vi "Exchange AI.vi"(8 "error in (no error)":errorcluster, 10 "AIP in":dbl[][](array[numeric]), 11 "AIP DVR":refnum<data-value>) -> (0 "error out":errorcluster, 2 "AIP out":dbl[][](array[numeric]), 3 "AIP DVR out":refnum<data-value>)   [LabVIEW 2019, in "Inputs.lvlib"]
uses:
  Inputs.lvlib
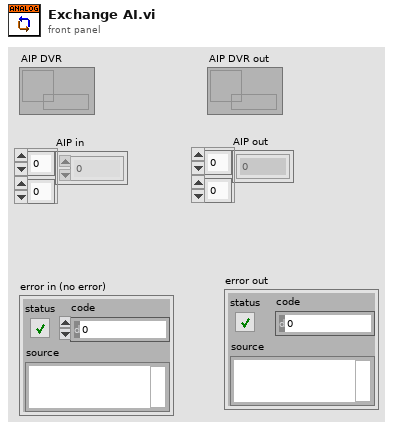
[diagram p1: front panel]
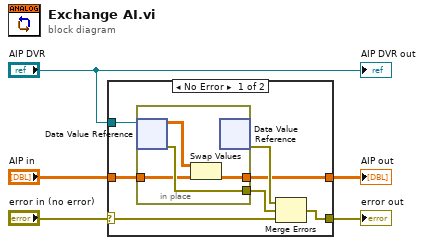
[diagram p0: block diagram]
diagram:
  n1 = case shown="No Error" "error in (no error)" {
    selector: "error in (no error)" -> [w10 w17]
    tunnel: [w8 w18] -> w5
    tunnel: "AIP in" -> [w9 w18]
    tunnel: "AIP DVR" -> [w7 _]
    tunnel: [w6 w17] -> w3
    frame No Error {
      n2 = in-place {
        in-place-border: [w16] -> w12
        in-place-border: w9 -> [w13]
        in-place-border: [w14] -> w8
        n3 = in-place-dvr #1(w7) -> (w15:dbl[][], w16:errorcluster)
        n4 = Swap Values(12:w15, 14:w13) -> (3:w14:dbl[][])  [unwired: 1 in, 1 out]
        n5 = in-place-dvr #1() -> (w11:errorcluster)  [unwired: 1 in, 1 out]
      }
      n6 = Merge Errors(w11, w12, w10) -> (w6:errorcluster)
    }
    frame Error {
    }
  }
  "AIP out" <- w5
  "error out" <- w3
  "AIP DVR out" <- "AIP DVR"
